vi "MatrixIO.vi"(1 "IOSource":T3={"Read (F)/ Write"=TRUE, "Path"=path "", "Datastream"="", "ArrayName"=""}, 2 "XArray in":dbl[](array[numeric]) caption="XArray" format="%.6f", 3 "YArray in":dbl[](array[numeric]) format="%.10e", 4 "ZMatrix in":dbl[][](array[numeric]) format="%.3f", 5 "error in":errorcluster, 6 "Header in":T2={"Separator"="\t", "Remarks"="", "NDim"=0}, 7 "Data names":T1) -> (12 "Header out":T2={"Separator"="\t", "Remarks"="", "NDim"=0}, 13 "Data names out":T1, 14 "Datastream out":string, 16 "XArray out":dbl[](array[numeric]) caption="XArray" format="%.6f", 17 "YArray out":dbl[](array[numeric]) format="%.10e", 18 "ZMatrix out":dbl[][](array[numeric]) format="%.3f", 19 "error out":errorcluster)   [LabVIEW 2026]
doc: "This VI reads or writes data files in matrix format. Sub-VI for 1D_Scan.vi, 2D_Scan.vi, Show_Save_Load_XY_Data.vi and Show_Save_Load_XYZ_Data.vi. See separate manual GCSData_User_SM146E.pdf and control descriptions in the diagram for more information."
uses:
  Support/GCSArray_regex_selector.ctl
  Support/GCSArray_regex_range.ctl
panel:
  out "Sample Time out":dbl format="%.10f"
  in  "Sample Time in":dbl format="%.10f"
  # "This vi reads or writes data files in matrix format. See separate manual \"GCSData User SM146E.pdf\" and control descriptions in the diagram for more information."
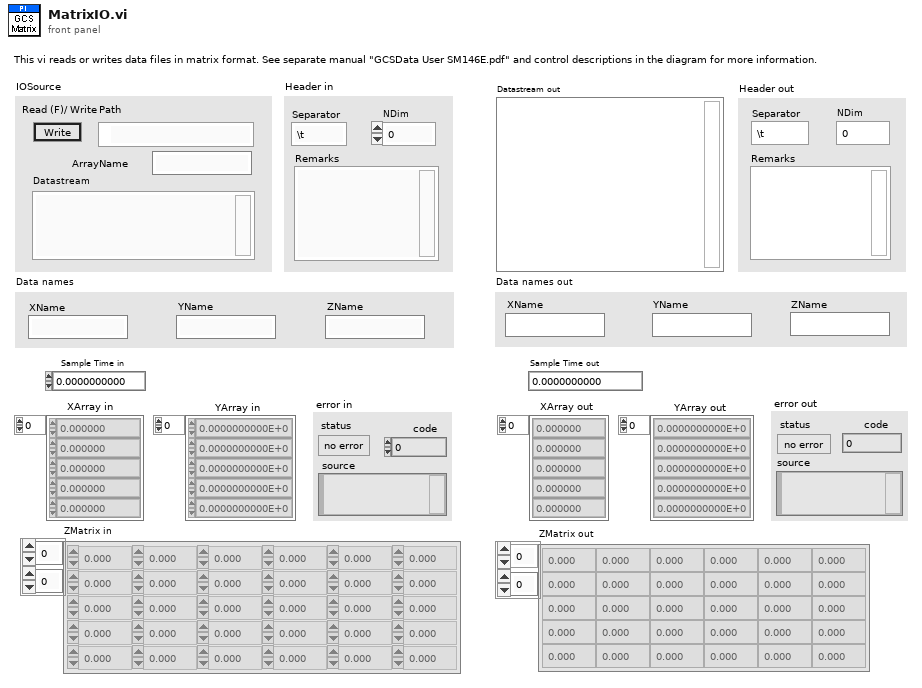
[diagram p1: front panel]
types:
  T1 = cluster{"XName":string, "YName":string, "ZName":string}
  T2 = cluster{"Separator":string, "Remarks":string, "NDim":i32}
  T3 = cluster{"Read (F)/ Write":bool, "Path":path, "Datastream":string, "ArrayName":string}
  T4 = enum16{"FirstTry", "Allocation", "FinalTry", "Native"}
  T5 = cluster{"separator":string, "remarks":string, "NDim":i32}
  T6 = typedef "GCSArray_regex_range.ctl" = cluster{"Begin":i32, "End":i32}
  T7 = typedef "GCSArray_regex_selector.ctl" = enum16{"GCS_ARRAY Block Full", "GCS_ARRAY Block ID", "GCS_ARRAY Block Header", "GCS_ARRAY Block Data", "GCS_ARRAY Identifier", "GCS_ARRAY Remark", "GCS_ARRAY Version", "GCS_ARRAY Dimension", "GCS_ARRAY Type", "GCS_ARRAY Separator", "GCS_ARRAY NData", "GCS_ARRAY NData%", "GCS_ARRAY NData% Keyword", "GCS_ARRAY Name%", "GCS_ARRAY Name% Keyword", "GCS_ARRAY Start%", "GCS_ARRAY Start% Keyword", "GCS_ARRAY End%", "GCS_ARRAY End% Keyword", "GCS_ARRAY Delta%", "GCS_ARRAY Delta% Keword", "GCS_ARRAY Sample Time", "GCS_ARRAY Unit of transmitted value%", "GCS_ARRAY Trans_Unit% Keyword", "GCS_ARRAY Trans_Unit% = RAW Keyword", "GCS_ARRAY Unit of displayed value%", "GCS_ARRAY Disp_Unit% Keyword", "GCS_ARRAY Nominator%", "GCS_ARRAY Ratio_Nom% Keyword", "GCS_ARRAY Denominator%", "GCS_ARRAY Ratio_Denom% Keyword", "GCS_ARRAY End of Header", "GCS_ARRAY Empty line of Header"}
  T8 = typedef "GCSArray_header.ctl" = cluster{"Identifier":string, "Version":i32, "Remark":string, "Dimension":i32, "Type":enum16{"Matrix", "Table"}, "Separator":u8, "NData":i32, "NData%":i32[], "Name%":string[], "Start%":dbl[], "End%":dbl[], "Delta%":dbl[], "SampleTime":dbl, "TransmittedUnit%":string[], "DisplayedUnit%":string[], "RatioNominator%":dbl[], "RatioDenominator%":dbl[]}
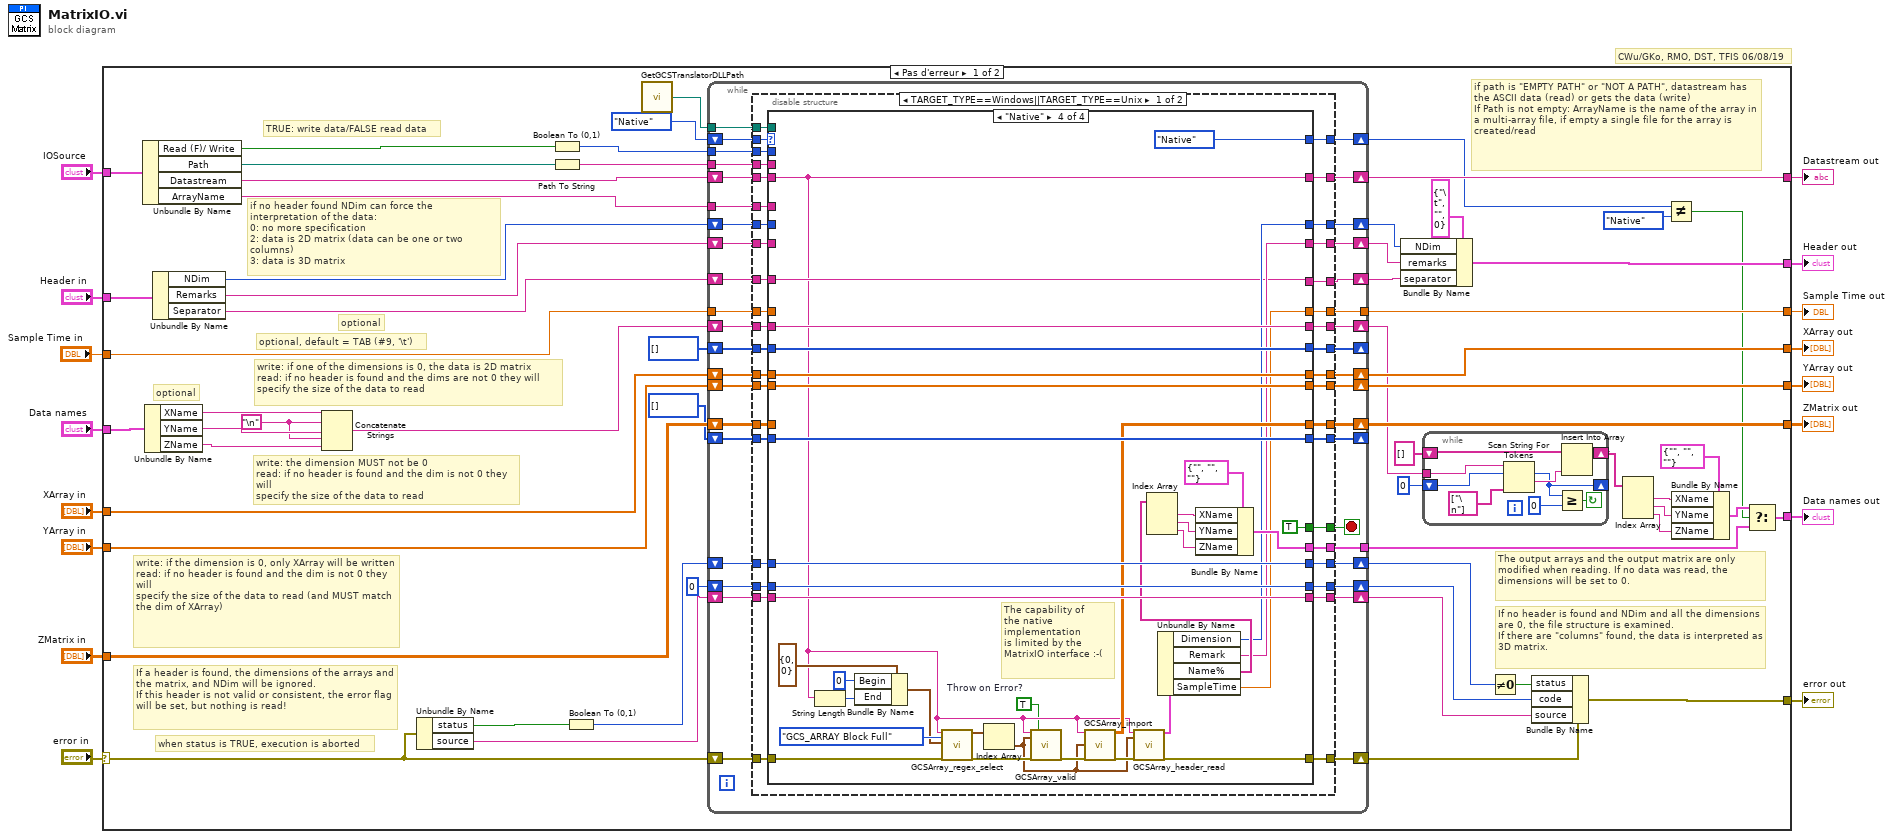
[diagram p0: block diagram]
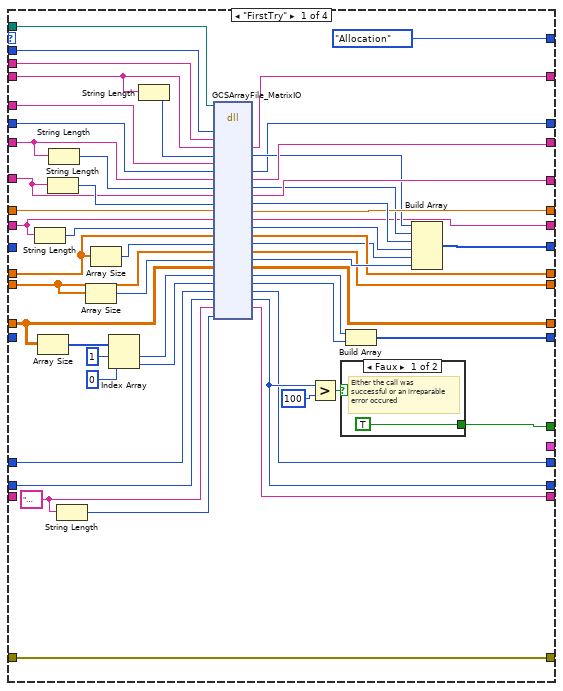
[diagram p2: hidden frame]
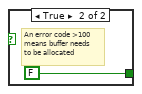
[diagram p3: hidden frame]
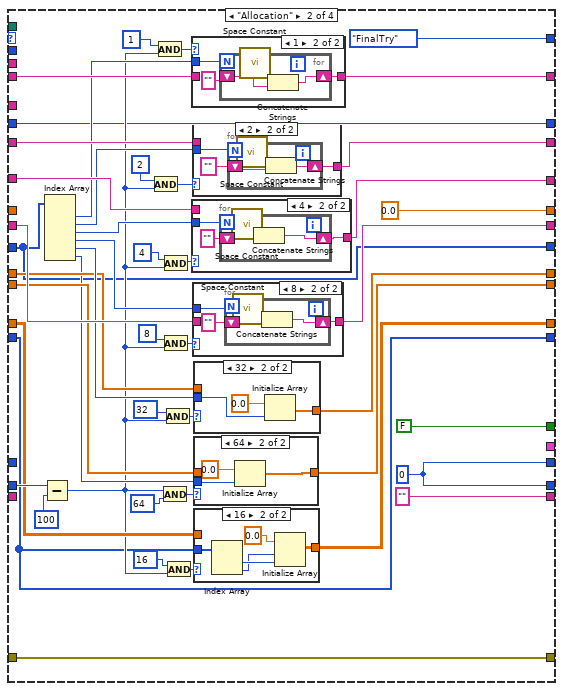
[diagram p4: hidden frame]
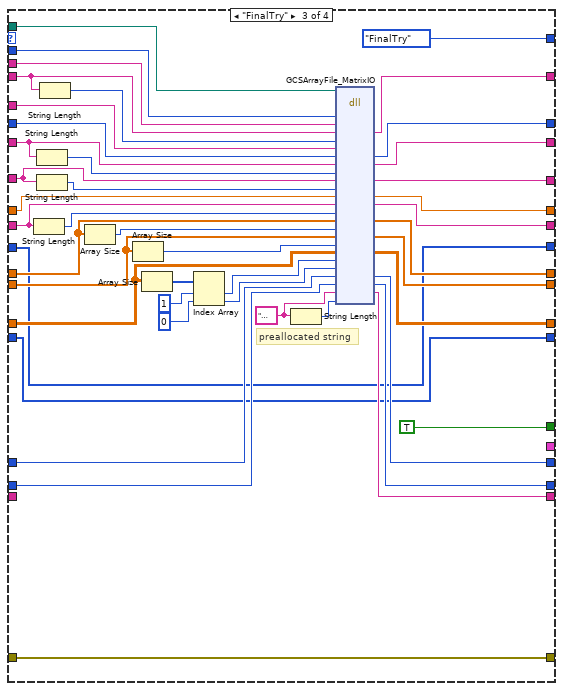
[diagram p12: hidden frame]
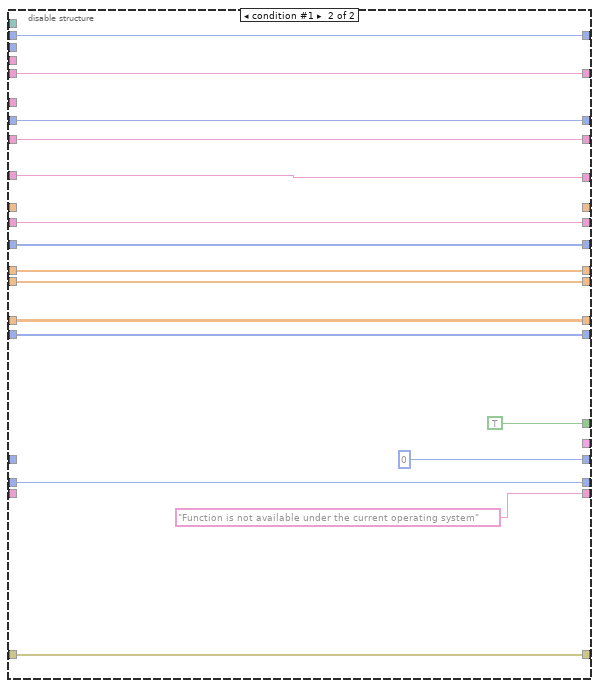
[diagram p13: hidden frame]
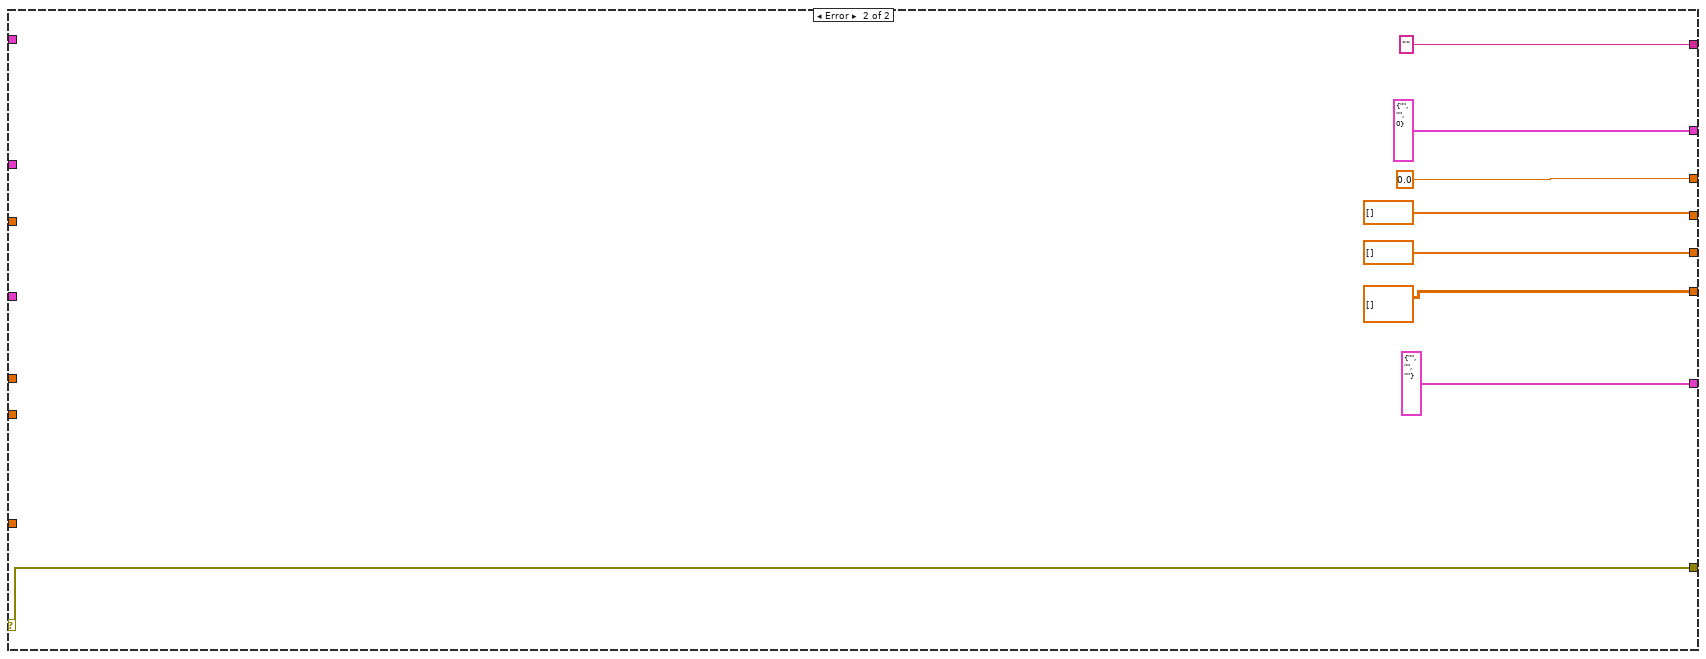
[diagram p14: hidden frame]
diagram:
  # "CWu/GKo, RMO, DST, TFIS 06/08/19"
  n1 = case shown="Pas d'erreur" "error in" {
    selector: "error in" -> [w24 w404]
    tunnel: "IOSource" -> [w76 _]
    tunnel: "Header in" -> [w75 _]
    tunnel: [w74 T5 {"separator"="", "remarks"="", "NDim"=0} ("header out")] -> w14
    tunnel: "Data names" -> [w73 _]
    tunnel: [w20 T1 {"XName"="", "YName"="", "ZName"=""} ("data out")] -> w12
    tunnel: [w68 w404] -> w11
    tunnel: [w34 0.0 ("Sample Time")] -> w10
    tunnel: [w64 "" ("DataStream")] -> w9
    tunnel: "Sample Time in" -> [w60 _]
    tunnel: "XArray in" -> [w59 _]
    tunnel: "YArray in" -> [w58 _]
    tunnel: "ZMatrix in" -> [w57 _]
    tunnel: [w49 dbl[] [] ("XArray")] -> w4
    tunnel: [w48 dbl[] [] ("YArray")] -> w3
    tunnel: [w47 dbl[][] [] ("ZMatrix")] -> w2
    frame No Error {
      w52 = "\n"
      # "The output arrays and the output matrix are only modified when reading. If no data was read, the dimensions will be set to 0."
      # "If no header is found and NDim and all the dimensions are 0, the file structure is examined.\nIf there are \"columns\" found, the data is interpreted as 3D matrix."
      # "If a header is found, the dimensions of the arrays and the matrix, and NDim will be ignored.\nIf this header is not valid or consistent, the error flag will be set, but nothing is read!"
      # "write: the dimension MUST not be 0\nread: if no header is found and the dim is not 0 they will\nspecify the size of the data to read"
      # "write: if the dimension is 0, only XArray will be written\nread: if no header is found and the dim is not 0 they will\nspecify the size of the data to read (and MUST match the dim of XArray)"
      # "write: if one of the dimensions is 0, the data is 2D matrix\nread: if no header is found and the dims are not 0 they will\nspecify the size of the data to read"
      # "when status is TRUE, execution is aborted"
      # "optional"
      # "optional, default = TAB (#9, '\\t')"
      # "optional"
      # "if no header found NDim can force the interpretation of the data:\n0: no more specification\n2: data is 2D matrix (data can be one or two columns)\n3: data is 3D matrix"
      # "if path is \"EMPTY PATH\" or \"NOT A PATH\", datastream has the ASCII data (read) or gets the data (write)\nIf Path is not empty: ArrayName is the name of the array in a multi-array file, if empty a single file for the array is created/read"
      # "TRUE: write data/FALSE read data"
      n2 = Unbundle By Name(w76) -> ("Read (F)/ Write"=w67:bool, "Path"=w70:path, "Datastream"=w61:string, "ArrayName"=w36:string)
      n3 = Unbundle By Name(w73) -> ("XName"=w54:string, "YName"=w53:string, "ZName"=w51:string)
      n4 = Unbundle By Name(w75) -> ("NDim"=w29:i32, "Remarks"=w27:string, "Separator"=w28:string)
      n5 = Concatenate Strings(w54, w52, w53, w52, w51) -> (w50:string)
      n6 = Unbundle By Name(w24) -> ("status"=w66:bool, "source"=w56:string)
      n7 = Boolean To (0,1)(Boolean=w67) -> (0, 1=w63:i16)
      n8 = Path To String(path=w70) -> (string=w62:string)
      n9 = Boolean To (0,1)(Boolean=w66) -> (0, 1=w55:i16)
      n10 = call "GetGCSTranslatorDLLPath.vi"() -> ("DLL path"=w30:path)  [unwired: 1 in]
      n11 = while {
        tunnel: w63 -> [w122]
        tunnel: w62 -> [w121]
        tunnel: w36 -> [w120]
        shift-right: [w114] -> w26
        shift-left: w29 -> [w118]
        shift-right: [w113] -> w25
        shift-left: w27 -> [w117]
        shift-right: [w112] -> w65
        shift-left: w28 -> [w116]
        shift-right: [w111] -> w47
        shift-left: w57 -> [w123]
        shift-right: [w109] -> w46
        shift-left: w55 -> [w115]
        shift-right: [w110] -> w45
        shift-left: 0 ("error code") -> [w107]
        shift-right: [w92] -> w21
        shift-left: T4."Native" -> [w91]
        shift-right: [w105] -> w64
        shift-left: w61 -> [w119]
        shift-right: [w93] -> w41
        shift-left: w50 -> [w102]
        shift-right: [w104] -> _
        shift-left: u32[] [] -> [w103]
        shift-right: [w101] -> _
        shift-left: u32[] [] -> [w100]
        shift-right: [w108] -> w44
        shift-left: w56 -> [w99]
        tunnel: w60 -> [w98]
        shift-right: [w95] -> w48
        shift-left: w58 -> [w96]
        shift-right: [w94] -> w49
        shift-left: w59 -> [w97]
        tunnel: [w90] -> w34
        tunnel: w30 -> [w89]
        shift-right: [w87] -> w23
        shift-left: w24 -> [w88]
        tunnel: [w86] -> w17
        stop <- w106 stop-if-true
        n12 = disable-structure shown="TARGET_TYPE==Windows||TARGET_TYPE==Unix" {
          disable-tunnel: w123 -> [w161 w401]
          disable-tunnel: w122 -> [w160 _]
          disable-tunnel: w121 -> [w159 _]
          disable-tunnel: w120 -> [w158 _]
          disable-tunnel: w119 -> [w157 w392]
          disable-tunnel: w118 -> [w156 w393]
          disable-tunnel: w117 -> [w155 w394]
          disable-tunnel: w116 -> [w154 w395]
          disable-tunnel: w115 -> [w153 _]
          disable-tunnel: [w152 w393] -> w114
          disable-tunnel: [w151 w394] -> w113
          disable-tunnel: [w150 w395] -> w112
          disable-tunnel: [w149 w401] -> w111
          disable-tunnel: [w148 w403] -> w110
          disable-tunnel: [w147 0 ("errorcode")] -> w109
          disable-tunnel: [w146 "Function is not available under the current operating system" ("error source")] -> w108
          disable-tunnel: w107 -> [w145 w403]
          disable-tunnel: [w144 TRUE] -> w106
          disable-tunnel: [w143 w392] -> w105
          disable-tunnel: [w142 w397] -> w104
          disable-tunnel: w103 -> [w141 w397]
          disable-tunnel: w102 -> [w140 w396]
          disable-tunnel: [w139 w400] -> w101
          disable-tunnel: w100 -> [w138 w400]
          disable-tunnel: w99 -> [w137 _]
          disable-tunnel: w98 -> [w136 _]
          disable-tunnel: w97 -> [w135 w398]
          disable-tunnel: w96 -> [w134 w399]
          disable-tunnel: [w133 w399] -> w95
          disable-tunnel: [w132 w398] -> w94
          disable-tunnel: [w131 w396] -> w93
          disable-tunnel: [w130 w391] -> w92
          disable-tunnel: w91 -> [w129 w391]
          disable-tunnel: [w128 _] -> w90
          disable-tunnel: w89 -> [w127 _]
          disable-tunnel: w88 -> [w126 w388]
          disable-tunnel: [w125 w388] -> w87
          disable-tunnel: [w124 _] -> w86
          frame condition #0 (active) {
            n13 = case shown="\"Native\"" w129 {
              tunnel: w161 -> [w179 w243 w336 _]
              tunnel: w160 -> [w194 _ w323 _]
              tunnel: w159 -> [w193 _ w347 _]
              tunnel: w158 -> [w190 _ w348 _]
              tunnel: w157 -> [w192 w258 w346 w353]
              tunnel: w156 -> [w189 w225 w342 _]
              tunnel: w155 -> [w188 w255 w344 _]
              tunnel: w154 -> [w185 w251 w339 w358]
              tunnel: w153 -> [w209 _ w328 w379]
              tunnel: [w173 w225 w341 w359] -> w152
              tunnel: [w195 w254 w330 w360] -> w151
              tunnel: [w196 w250 w331 w358] -> w150
              tunnel: [w204 w244 w334 w369] -> w149
              tunnel: [w207 w221 w326 w380] -> w148
              tunnel: [w206 w221 w327 w379] -> w147
              tunnel: [w208 "" ("errorsource") w325 w381] -> w146
              tunnel: w145 -> [w211 w263 w324 w380]
              tunnel: [w166 FALSE TRUE TRUE] -> w144
              tunnel: [w172 w259 w329 w353] -> w143
              tunnel: [w214 w222 w312 w375] -> w142
              tunnel: w141 -> [_ w222 w312 w375]
              tunnel: w140 -> [w183 w247 w318 w374]
              tunnel: [w215 w220 w311 w378] -> w139
              tunnel: w138 -> [_ w220 w311 w378]
              tunnel: w137 -> [_ _ _ w381]
              tunnel: [w202 w229 w333 w377] -> w133
              tunnel: [w201 w228 w317 w376] -> w132
              tunnel: [w197 0.0 ("Sample Time") w332 w361] -> w128
              tunnel: w136 -> [w184 _ w338 _]
              tunnel: w135 -> [w181 w234 w321 w376]
              tunnel: w134 -> [w177 w233 w335 w377]
              tunnel: [w171 w227 w322 w374] -> w131
              tunnel: [T4."Allocation" T4."FinalTry" T4."FinalTry" T4."Native"] -> w130
              tunnel: w127 -> [w164 _ w310 _]
              tunnel: w126 -> [w162 w219 w307 w383]
              tunnel: [w162 w219 w307 w357] -> w125
              tunnel: [_ _ _ w363] -> w124
              frame "FirstTry" {
                w163 = "                                                                                                                                             " ("string")
                n14 = String Length(string=w183) -> (length=w182:i32)
                n15 = Array Size(array=w179) -> (size(s)=w216:i32[])
                n16 = String Length(string=w185) -> (length=w186:i32)
                n17 = String Length(string=w188) -> (length=w187:i32)
                n18 = String Length(string=w163) -> (length=w210:i32)
                n19 = Array Size(array=w177) -> (size(s)=w178:i32)
                n20 = Array Size(array=w181) -> (size(s)=w180:i32)
                n21 = Index Array(array=w216, index #1=1 ("index"), index #2=0 ("index")) -> (element #1=w168:i32, element #2=w167:i32)
                n22 = String Length(string=w192) -> (length=w191:i32)
                n23 = dll-call lib="T:/Entwicklung/HostSoftware/LabVIEW/GCSDrivers/source/GCS2LabVIEW/Low Level/GCSTranslator.dll" fn="GCSArrayFile_MatrixIO" ("GCSTranslator.dll:GCSArrayIO")(path in=w164, "WriteAccess"=w194, "Path"=w193, "DataStream"=w192, "DataStreamBufferSize"=w191, "ArrayName"=w190, "NDim"=w189, "Remarks"=w188, "RemarksBufferSize"=w187, "Separator"=w185, "SeparatorBufferSize"=w186, "Sample Time"=w184, "Names"=w183, "NamesBufferSize"=w182, "XArray"=w181, "XArray size"=w180, "YArray"=w177, "YArray size"=w178, "ZMatrix"=w179, "ZMatrixNColumns"=w168, "ZMatrixNRows"=w167, "error state"=w209, "error code"=w211, "error source"=w163, "errorsrcbuflen"=w210) -> ("DataStream"=w172:string, "DataStreamBufferSize"=w174:u32, "NDim"=w173:i32, "Remarks"=w195:string, "RemarksBufferSize"=w175:u32, "Separator"=w196:string, "SeparatorBufferSize"=w198:u32, "Sample Time"=w197:dbl, "Names"=w171:string, "NamesBufferSize"=w199:u32, "XArray"=w201:dbl[], "XArray size"=w200:u32, "YArray"=w202:dbl[], "YArray size"=w203:u32, "ZMatrix"=w204:dbl[][], "ZMatrixNColumns"=w176:u32, "ZMatrixNRows"=w205:u32, "error state"=w206:u8, "error code"=w207:i32, "error source"=w208:string)  [unwired: 5 in, 4 out]
                n24 = Greater?(x=w207, y=100 ("x")) -> (0:w213:bool)
                n25 = case shown="Faux" w213 {
                  tunnel: [TRUE FALSE] -> w166
                  frame False {
                    # "Either the call was\nsuccessful or an irreparable\nerror occured"
                  }
                  frame True {
                    # "An error code >100\nmeans buffer needs\nto be allocated"
                  }
                }
                n26 = Build Array(w176, w205) -> (w215:u32[])
                n27 = Build Array(w174, w175, w198, w199, w200, w203) -> (w214:u32[])
              }
              frame "Allocation" {
                w221 = 0 ("errorcode")
                n28 = Subtract(x=w263, y=100) -> (x-y=w226:i32)
                n29 = Index Array(array=w222) -> (element #1=w239:u32, element #2=w240:u32, element #3=w241:u32, element #4=w236:u32, element #5=w235:u32, element #6=w232:u32)  [unwired: 6 in]
                n30 = And(x=2, y=w226) -> (x .and. y?=w257:i32)
                n31 = And(x=1, y=w226) -> (x .and. y?=w260:i32)
                n32 = And(x=w226, y=64 ("x")) -> (x .and. y?=w231:i32)
                n33 = And(x=4, y=w226) -> (x .and. y?=w253:i32)
                n34 = And(x=8, y=w226) -> (x .and. y?=w249:i32)
                n35 = And(x=32, y=w226) -> (x .and. y?=w237:i32)
                n36 = And(x=16, y=w226) -> (x .and. y?=w246:i32)
                n37 = case shown="1" w260 {
                  tunnel: [w300 w302] -> w259
                  tunnel: w258 -> [w300 _]
                  tunnel: w239 -> [_ w301]
                  frame 0, Default {
                  }
                  frame 1 {
                    n38 = for {
                      N: w301 -> [_]
                      shift-right: [w305] -> w302
                      shift-left: "" -> [w304]
                      n39 = call <vilib>:"Space Constant.vi"() -> ("String"=w306:string)
                      n40 = Concatenate Strings(w306, w304) -> (w305:string)
                    }
                  }
                }
                n41 = case shown="4" w253 {
                  tunnel: [w286 w288] -> w250
                  tunnel: w251 -> [w286 _]
                  tunnel: w241 -> [_ w287]
                  frame 0, Default {
                  }
                  frame 4 {
                    n42 = for {
                      N: w287 -> [_]
                      shift-right: [w291] -> w288
                      shift-left: "" -> [w290]
                      n43 = call <vilib>:"Space Constant.vi"() -> ("String"=w292:string)
                      n44 = Concatenate Strings(w292, w290) -> (w291:string)
                    }
                  }
                }
                n45 = case shown="2" w257 {
                  tunnel: [w293 w295] -> w254
                  tunnel: w255 -> [w293 _]
                  tunnel: w240 -> [_ w294]
                  frame 0, Default {
                  }
                  frame 2 {
                    n46 = for {
                      N: w294 -> [_]
                      shift-right: [w298] -> w295
                      shift-left: "" -> [w297]
                      n47 = call <vilib>:"Space Constant.vi"() -> ("String"=w299:string)
                      n48 = Concatenate Strings(w299, w297) -> (w298:string)
                    }
                  }
                }
                n49 = case shown="8" w249 {
                  tunnel: [w279 w281] -> w227
                  tunnel: w247 -> [w279 _]
                  tunnel: w236 -> [_ w280]
                  frame 0, Default {
                  }
                  frame 8 {
                    n50 = for {
                      N: w280 -> [_]
                      shift-right: [w284] -> w281
                      shift-left: "" -> [w283]
                      n51 = call <vilib>:"Space Constant.vi"() -> ("String"=w285:string)
                      n52 = Concatenate Strings(w285, w283) -> (w284:string)
                    }
                  }
                }
                n53 = case shown="32" w237 {
                  tunnel: [w269 w272] -> w228
                  tunnel: w234 -> [w269 _]
                  tunnel: w235 -> [_ w270]
                  frame 0, Default {
                  }
                  frame 32 {
                    n54 = Initialize Array(0.0 ("element"), w270) -> (w272:dbl[])
                  }
                }
                n55 = case shown="64" w231 {
                  tunnel: [w265 w268] -> w229
                  tunnel: w233 -> [w265 _]
                  tunnel: w232 -> [_ w266]
                  frame 0, Default {
                  }
                  frame 64 {
                    n56 = Initialize Array(0.0 ("element"), w266) -> (w268:dbl[])
                  }
                }
                n57 = case shown="16" w246 {
                  tunnel: [w273 w278] -> w244
                  tunnel: w243 -> [w273 _]
                  tunnel: w220 -> [_ w276]
                  frame 0, Default {
                  }
                  frame 16 {
                    n58 = Index Array(array=w276) -> (element #1=w275:u32, element #2=w274:u32)  [unwired: 2 in]
                    n59 = Initialize Array(0.0 ("element"), w274, w275) -> (w278:dbl[][])
                  }
                }
              }
              frame "FinalTry" {
                w309 = "                                                                                                                                             " ("string")
                # "preallocated string"
                n60 = String Length(string=w318) -> (length=w319:i32)
                n61 = String Length(string=w344) -> (length=w343:i32)
                n62 = String Length(string=w339) -> (length=w340:i32)
                n63 = String Length(string=w346) -> (length=w345:i32)
                n64 = Array Size(array=w321) -> (size(s)=w320:i32)
                n65 = Array Size(array=w335) -> (size(s)=w337:i32)
                n66 = Array Size(array=w336) -> (size(s)=w351:i32[])
                n67 = Index Array(array=w351, index #1=1 ("index"), index #2=0 ("index")) -> (element #1=w315:i32, element #2=w314:i32)
                n68 = String Length(string=w309) -> (length=w349:i32)
                n69 = dll-call lib="T:/Entwicklung/HostSoftware/LabVIEW/GCSDrivers/source/GCS2LabVIEW/Low Level/GCSTranslator.dll" fn="GCSArrayFile_MatrixIO" ("GCSTranslator.dll:GCSArrayIO")(path in=w310, "WriteAccess"=w323, "Path"=w347, "DataStream"=w346, "DataStreamBufferSize"=w345, "ArrayName"=w348, "NDim"=w342, "Remarks"=w344, "RemarksBufferSize"=w343, "Separator"=w339, "SeparatorBufferSize"=w340, "Sample Time"=w338, "Names"=w318, "NamesBufferSize"=w319, "XArray"=w321, "XArray size"=w320, "YArray"=w335, "YArray size"=w337, "ZMatrix"=w336, "ZMatrixNColumns"=w315, "ZMatrixNRows"=w314, "error state"=w328, "error code"=w324, "error source"=w309, "errorsrcbuflen"=w349) -> ("DataStream"=w329:string, "NDim"=w341:i32, "Remarks"=w330:string, "Separator"=w331:string, "Sample Time"=w332:dbl, "Names"=w322:string, "XArray"=w317:dbl[], "YArray"=w333:dbl[], "ZMatrix"=w334:dbl[][], "error state"=w327:u8, "error code"=w326:i32, "error source"=w325:string)  [unwired: 12 in, 5 out]
              }
              frame "Native" {
                w352 = TRUE  # Throw on Error?
                # "The capability of\nthe native\nimplementation\nis limited by the\nMatrixIO interface :-("
                n70 = String Length(string=w353) -> (length=w371:i32)
                n71 = Bundle By Name(cluster=T6 {"Begin"=0, "End"=0} ("Range"), "Begin"=0, "End"=w371) -> (w370:T6)
                n72 = call "GCSArray_regex_select.vi"("GCSArray input string"=w353, "Selector"=GCSArray_regex_selector."GCS_ARRAY Block Full", "Range"=w370, "error in (no error)"=w383) -> ("Matches"=w385:T6[], "error out"=w356:errorcluster)  [unwired: 14 out]
                n73 = Index Array(array=w385) -> (element=w354:T6)  [unwired: 1 in]
                n74 = call "GCSArray_valid.vi"("GCSArray input string"=w353, "Selection"=w354, "error in (no error)"=w356, "Throw on Error?"=w352) -> ("error out"=w355:errorcluster)  [unwired: 15 out]
                n75 = call "GCSArray_import.vi"("GCSArray input string"=w353, "Range"=w354, "error in (no error)"=w355) -> ("GCSArray data"=w369:dbl[][], "error out"=w382:errorcluster)  [unwired: 15 out]
                n76 = call "GCSArray_header_read.vi"("GCSArray input string"=w353, "Range"=w354, "error in (no error)"=w382) -> ("GCSArray Header"=w368:T8, "error out"=w357:errorcluster)  [unwired: 15 out]
                n77 = Unbundle By Name(w368) -> ("Dimension"=w359:i32, "Remark"=w360:string, "Name%"=w362:string[], "SampleTime"=w361:dbl)
                n78 = Index Array(array=w362) -> (element #1=w366:string, element #2=w365:string, element #3=w364:string)  [unwired: 3 in]
                n79 = Bundle By Name(cluster=T1 {"XName"="", "YName"="", "ZName"=""} ("data out"), "XName"=w366, "YName"=w365, "ZName"=w364) -> (w363:T1)
              }
            }
          }
          frame condition #1 {
          }
        }
      }
      n80 = Bundle By Name(cluster=T5 {"separator"="\t", "remarks"="", "NDim"=0} ("header out"), "NDim"=w26, "remarks"=w25, "separator"=w65) -> (w74:T5)
      n81 = while {
        shift-right: [w83] -> w40
        shift-left: string[] [] -> [w82]
        shift-right: [w79] -> _
        shift-left: 0 ("offset past token") -> [w80]
        tunnel: w41 -> [w78]
        stop <- w84 continue-if-true
        n82 = Scan String For Tokens(6:string[] ["\n"] ("delimiters (\\s,\\t,\\r,\\n)"), 8:w80, 9:w78) -> (1:w81:string, 2:w79:i32)  [unwired: 5 out]
        n83 = Greater Or Equal?(x=w79, y=0) -> (x >= y?=w84:bool)
        n84 = Insert Into Array(array=w82, new element=w81) -> (w83:string[])  [unwired: 1 in]
      }
      n85 = Not Equal To 0?(x=w46) -> (x != 0?=w69:bool)
      n86 = Bundle By Name(cluster=w23, "status"=w69, "code"=w45, "source"=w44) -> (w68:errorcluster)
      n87 = Index Array(array=w40) -> (element #1=w39:string, element #2=w38:string, element #3=w37:string)  [unwired: 3 in]
      n88 = Not Equal?(x=w21, y=T4."Native") -> (x != y?=w18:bool)
      n89 = Bundle By Name(cluster=T1 {"XName"="", "YName"="", "ZName"=""} ("data out"), "XName"=w39, "YName"=w38, "ZName"=w37) -> (w19:T1)
      n90 = Select(t=w19, s=w18, f=w17) -> (s? t:f=w20:T1)
    }
    frame Error {
    }
  }
  "error out" <- w11
  "Datastream out" <- w9
  "Header out" <- w14
  "Data names out" <- w12
  "XArray out" <- w4
  "YArray out" <- w3
  "ZMatrix out" <- w2
  "Sample Time out" <- w10
